vi "GUNSC_GetPhysMap.vi"(10 "Database RefNum in":T1, 11 "num amps":u16=128) -> (2 "response":string)   [LabVIEW 2016]
uses:
  DBSHAND/private/vis/DatabaseHand_RefNum.ctl
  DBSHAND/private/vis/DatabaseHand_Element_Get(1DArr).vi
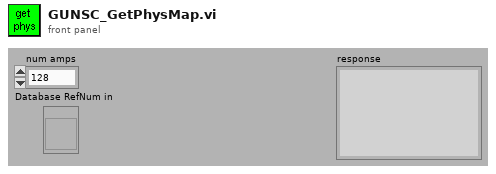
[diagram p1: front panel]
types:
  T1 = typedef "DatabaseHand_RefNum.ctl" = refnum<vi>
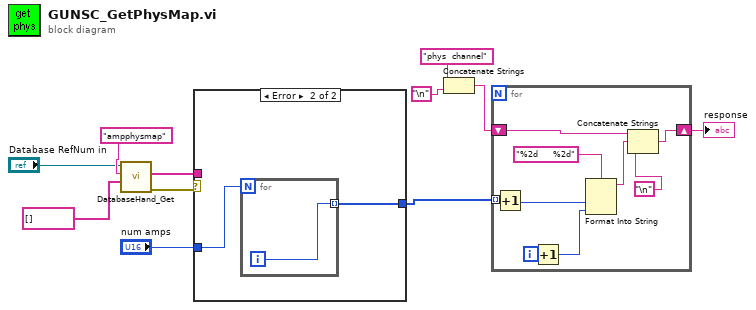
[diagram p0: block diagram]
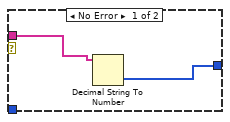
[diagram p2: hidden frame]
diagram:
  n1 = call-poly "DatabaseHand_Get.vi"("default value"=string[] [], "name"="ampphysmap", "Database RefNum in"="Database RefNum in") -> ("error out"=w9:errorcluster, "value"=w7:string[])  [unwired: 2 in, 5 out]
  n2 = case shown="Error" w9 {
    tunnel: "num amps" -> [_ w15]
    tunnel: w7 -> [w13 _]
    tunnel: [w12 w14] -> w1
    frame No Error {
      n3 = Decimal String To Number(string=w13) -> (number=w12:i32[])  [unwired: 3 out]
    }
    frame Error {
      n4 = for {
        N: w15 -> [_]
        tunnel: [w16] -> w14 mode=indexing
        i -> [w16]
      }
    }
  }
  n5 = Concatenate Strings("phys  channel", "\n") -> (w4:string)
  n6 = for {
    shift-right: [w20] -> w3
    shift-left: w4 -> [w23]
    tunnel: w1 -> [w19] mode=indexing
    i -> [w25]
    n7 = Increment(x=w19) -> (x+1=w18:i32)
    n8 = Increment(x=w25) -> (x+1=w17:i32)
    n9 = Format Into String(format string="%2d     %2d", w18, w17) -> (resulting string=w22:string)  [unwired: 2 in, 1 out]
    n10 = Concatenate Strings(w23, w22, "\n") -> (w20:string)
  }
  "response" <- w3
